vi "7813r01.vi"() -> ()   [LabVIEW 2018]
uses:
  <vilib>/Platform/TimedLoop/XDataNode/timing_clust.ctl
  <vilib>/Platform/TimedLoop/XDataNode/nitl_modes.ctl
  <vilib>/Platform/TimedLoop/XDataNode/wakeup.ctl
  <vilib>/rvi/Emulation/niFpgaGetClockAttributes.vi
  <vilib>/rvi/Emulation/niFpgaSctlEmulationGetInTimedLoop.vi
  <vilib>/rvi/Emulation/niFpgaEmulationReportErrorSimple.vi
  <vilib>/rvi/Emulation/niFpgaProcessEmulError.vi
  <vilib>/rvi/Emulation/niFpgaCriticalErrorInLSC.vi
  <vilib>/rvi/eio/common/nirviEmuTemplateMethod_errors.vi
  <vilib>/Platform/TimedLoop/XDataNode/XDataNode.xnode
  <vilib>/eio/EIONode/EIONode.xnode
  <vilib>/Platform/TimedLoop/XDataNode/XDNodeRunTimeDep.lvlib
panel:
  out "act":bool[](array[boolean])
  out "width":i32[](array[numeric])
  out "begin":i32[](array[numeric])
  in  "禁用shutup":bool
  in  "禁用trigger":bool
  out "T-run":bool
  in  "ShutUp":bool
  in  "Ready":bool
  in  "Abort":bool
  in  "max0+1":u32
  out "stop":bool
  in  "running":bool
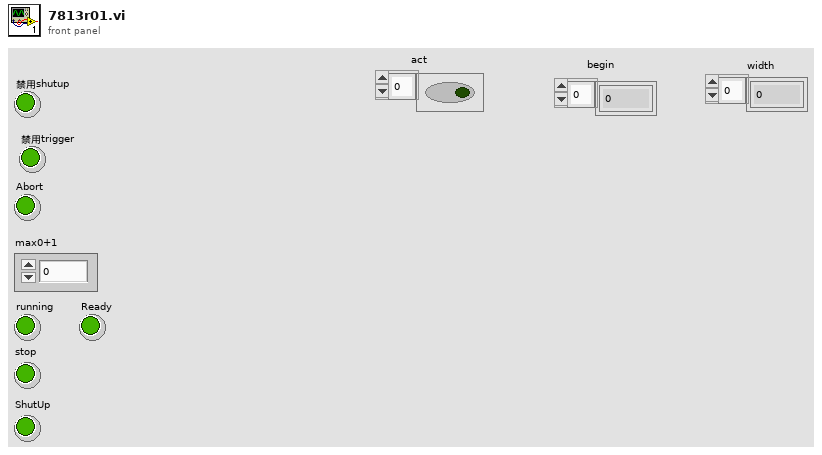
[diagram p1: front panel]
types:
  T1 = typedef "XDNodeRunTimeDep.lvlib/timing_clust.ctl" = cluster{"Expected End [f-1]":u64, "Actual End [f-1]":u64, "Finished Late? [f-1]":bool, "Expected End [i-1]":u64, "Actual End [i-1]":u64, "Finished Late? [i-1]":bool, "Expected Start [i]":u64, "Actual Start [i]":u64, "Expected Start [f]":u64, "Actual Start [f]":u64, "Source Name":string, "Structure Name":string, "Period":i64, "Deadline":i64, "Offset":i64, "Start":i64, "Priority":i32, "Timeout":i32, "Mode":T2, "Wakeup Reason":T3, "Error":errorcluster, "Source Type":string, "Secondary Source Type":string, "Global End Time":u64, "Global Start Time":u64, "Frame Duration":u64, "Iteration Duration":u64, "Assigned CPU":i32, "I/O Scan Engine Mode":u32}
  T2 = typedef "XDNodeRunTimeDep.lvlib/nitl_modes.ctl" = enum32{"No Change", "Process missed periods, maintain original phase", "Discard missed periods, maintain original phase", "Process missed periods, ignore original phase", "Discard missed periods, ignore original phase"}
  T3 = typedef "XDNodeRunTimeDep.lvlib/wakeup.ctl" = enum32{"Normal", "Aborted", "Asynchronous wakeup", "Timing source error", "Timed loop error", "Timeout"}
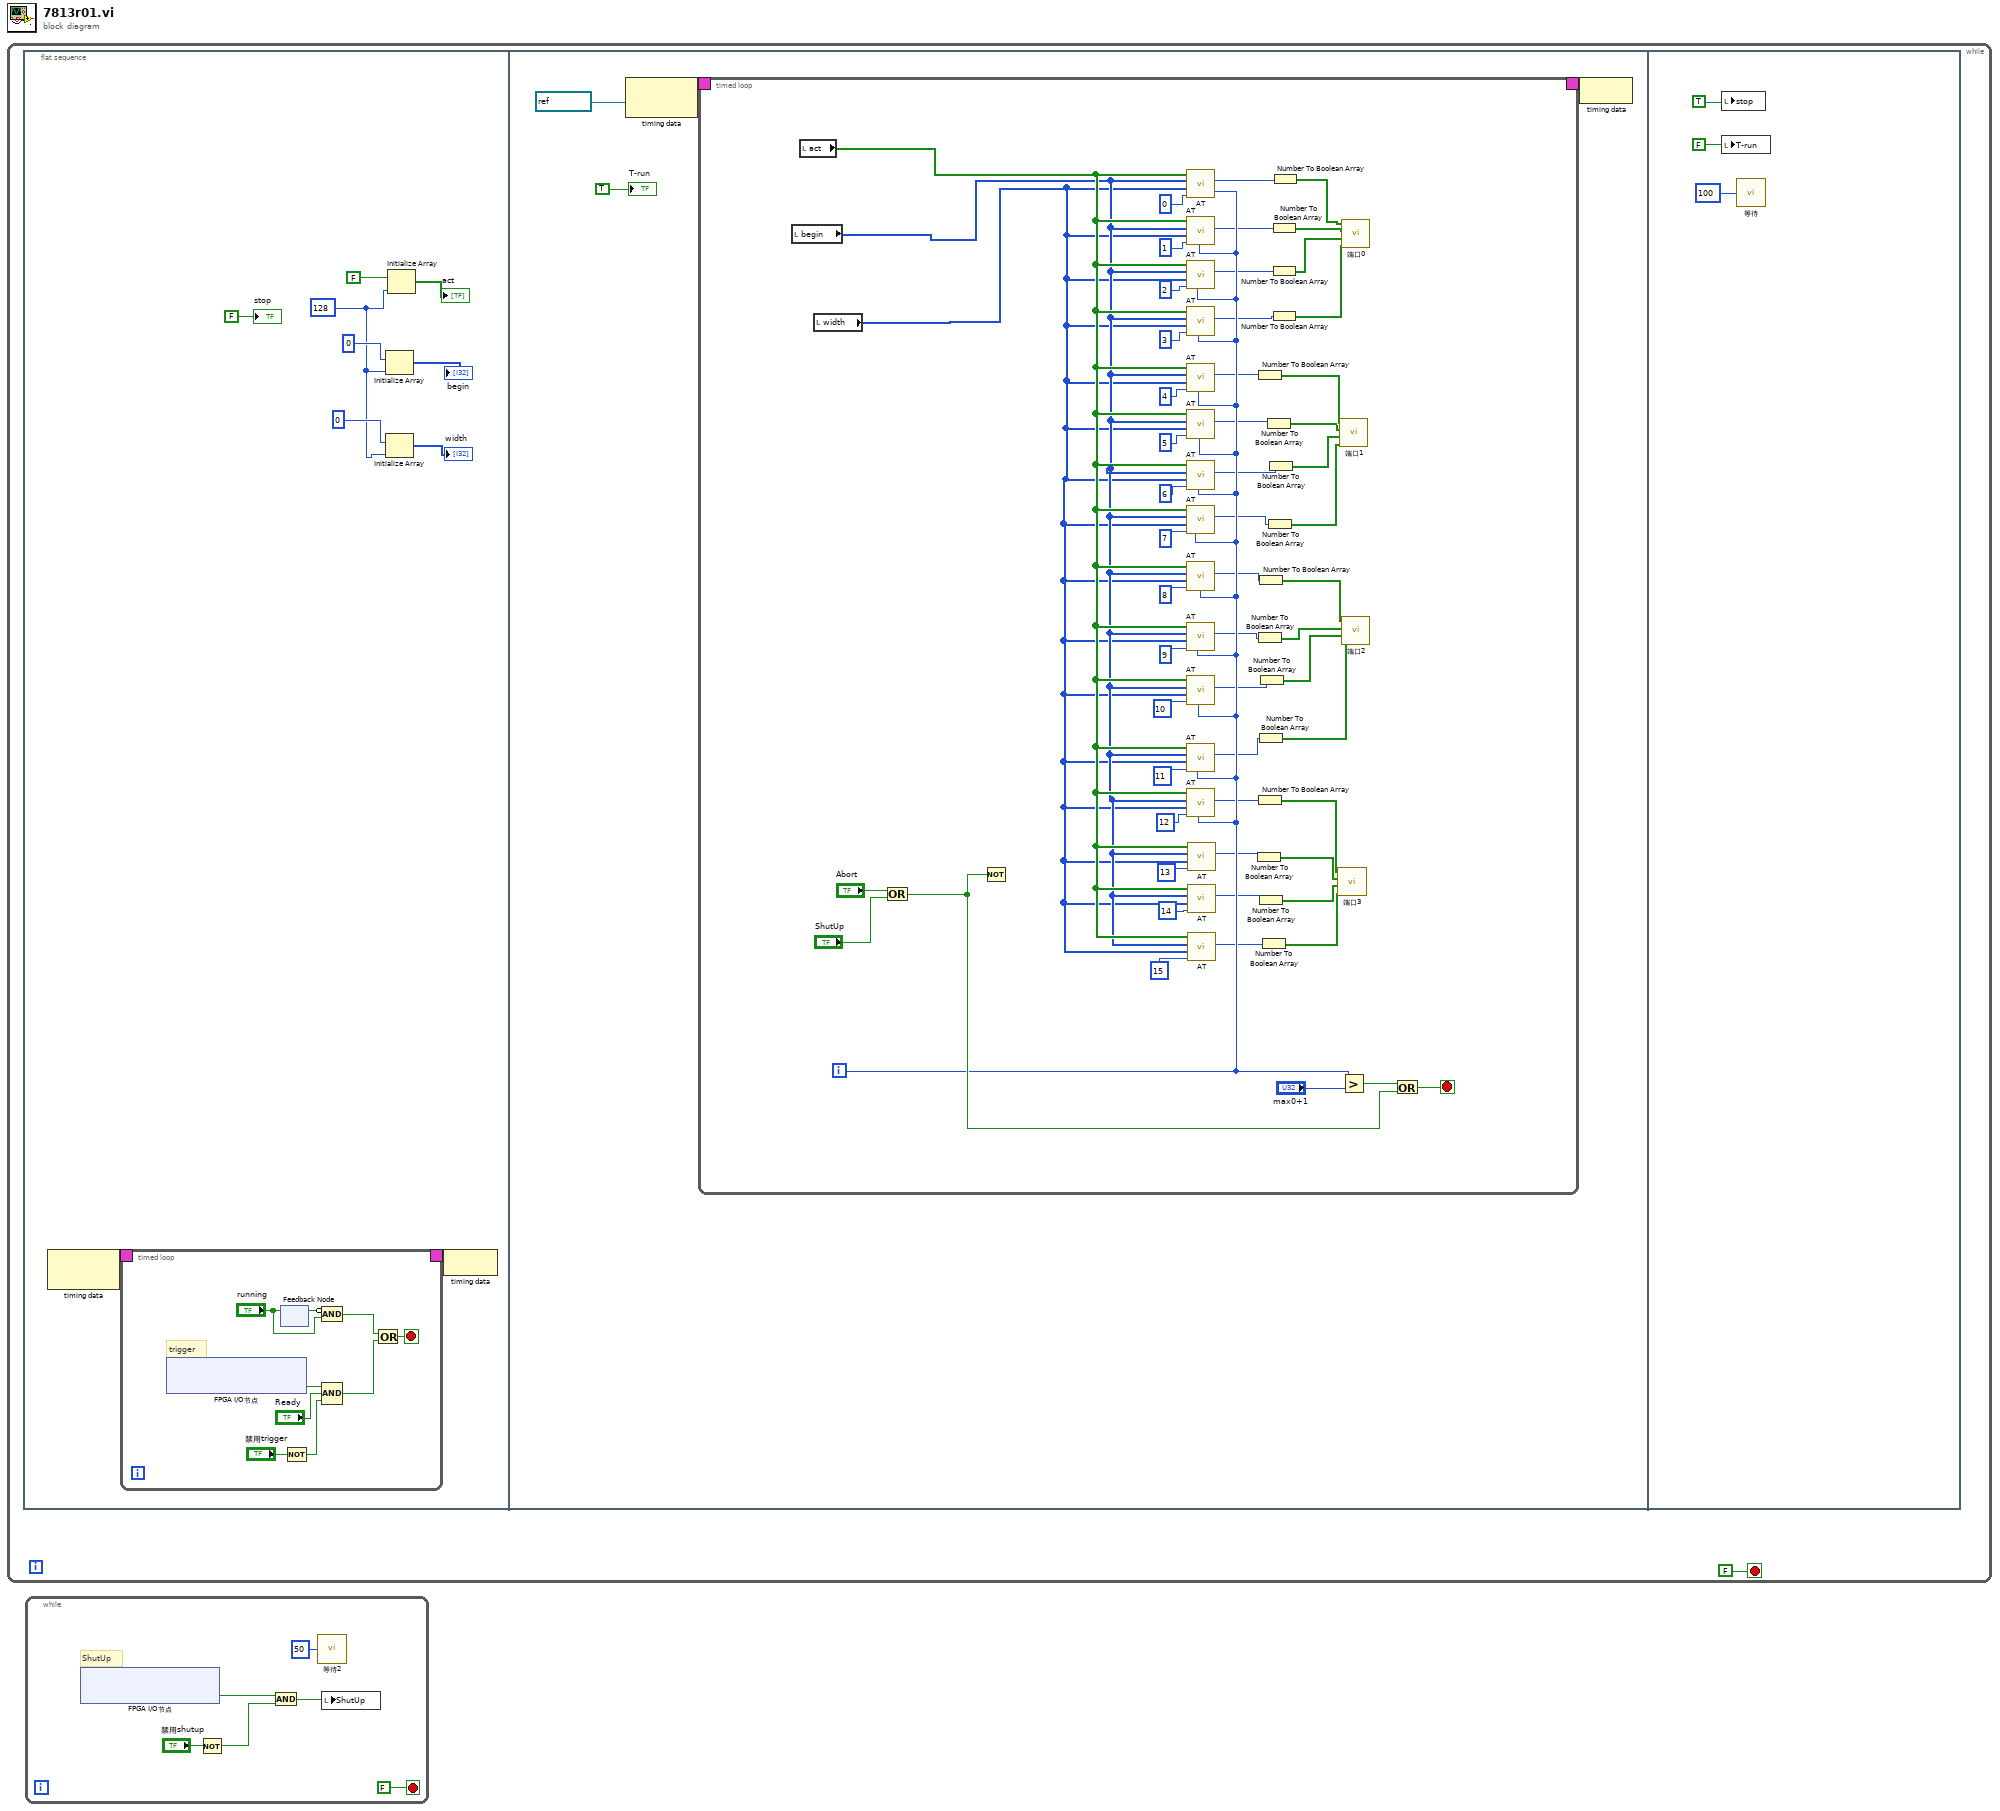
[diagram p0: block diagram]
diagram:
  n1 = while {
    stop <- FALSE stop-if-true
    n2 = flat-sequence {
      frame #0 {
        w2 = i16 128
        n3 = node-c288() -> (w11:T1)  [unwired: 1 in]
        n4 = timed-loop {
          timing: w11 -> [_]
          timing-out: [_] -> w10
          stop <- w19 stop-if-true
          # "trigger"
          n5 = xnode "FPGA I/O节点"() -> ("Connector0/DIO38"=w12:bool)  [unwired: 1 in, 1 out]
          n6 = feedback #1() -> (w15:bool)  [unwired: 1 in]
          n7 = feedback-in #1("running") -> ()
          n8 = Not(x="禁用trigger") -> (.not. x?=w16:bool)
          n9 = Compound Arithmetic op=AND(invert w15, "running") -> (w13:bool)
          n10 = Compound Arithmetic op=AND(w12, "Ready", w16) -> (w18:bool)
          n11 = Or(x=w13, y=w18) -> (x .or. y?=w19:bool)
        }
        n12 = Initialize Array(i16 0, w2) -> (→"begin":i16[])
        n13 = Initialize Array(i16 0, w2) -> (→"width":i16[])
        n14 = Initialize Array(FALSE, w2) -> (→"act":bool[])
        n15 = node-c288(w10) -> ()
        "stop" <- FALSE ("running")
      }
      frame #1 {
        n16 = node-c288(refnum<k21> "5MHz" ("源名称")) -> (w28:T1)
        n17 = timed-loop {
          timing: w28 -> [_]
          timing-out: [_] -> w27
          i -> [w67]
          stop <- w84 stop-if-true
          n18 = local read "begin"() -> (w62:i32[])
          n19 = local read "act"() -> (w63:bool[])
          n20 = local read "width"() -> (w61:i32[])
          n21 = Or(x="Abort", y="ShutUp") -> (x .or. y?=w83:bool)
          n22 = Not(x=w83) -> ()  [unwired: 1 out]
          n23 = call "AT.vi"("时间值"=w67, "数值"=i16 0, "width"=w61, "begin"=w62, "act"=w63) -> ("数字"=w60:u8)  [unwired: 6 in]
          n24 = call "AT.vi"("时间值"=w67, "数值"=i16 1, "width"=w61, "begin"=w62, "act"=w63) -> ("数字"=w59:u8)  [unwired: 6 in]
          n25 = call "AT.vi"("时间值"=w67, "数值"=i16 2, "width"=w61, "begin"=w62, "act"=w63) -> ("数字"=w58:u8)  [unwired: 6 in]
          n26 = call "AT.vi"("时间值"=w67, "数值"=i16 3, "width"=w61, "begin"=w62, "act"=w63) -> ("数字"=w57:u8)  [unwired: 6 in]
          n27 = call "AT.vi"("时间值"=w67, "数值"=i16 4, "width"=w61, "begin"=w62, "act"=w63) -> ("数字"=w52:u8)  [unwired: 6 in]
          n28 = call "AT.vi"("时间值"=w67, "数值"=i16 5, "width"=w61, "begin"=w62, "act"=w63) -> ("数字"=w51:u8)  [unwired: 6 in]
          n29 = call "AT.vi"("时间值"=w67, "数值"=i16 6, "width"=w61, "begin"=w62, "act"=w63) -> ("数字"=w50:u8)  [unwired: 6 in]
          n30 = call "AT.vi"("时间值"=w67, "数值"=i16 7, "width"=w61, "begin"=w62, "act"=w63) -> ("数字"=w49:u8)  [unwired: 6 in]
          n31 = call "AT.vi"("时间值"=w67, "数值"=i16 8, "width"=w61, "begin"=w62, "act"=w63) -> ("数字"=w44:u8)  [unwired: 6 in]
          n32 = call "AT.vi"("时间值"=w67, "数值"=i16 9, "width"=w61, "begin"=w62, "act"=w63) -> ("数字"=w43:u8)  [unwired: 6 in]
          n33 = call "AT.vi"("时间值"=w67, "数值"=i16 10, "width"=w61, "begin"=w62, "act"=w63) -> ("数字"=w42:u8)  [unwired: 6 in]
          n34 = call "AT.vi"("时间值"=w67, "数值"=i16 11, "width"=w61, "begin"=w62, "act"=w63) -> ("数字"=w41:u8)  [unwired: 6 in]
          n35 = call "AT.vi"("时间值"=w67, "数值"=i16 12, "width"=w61, "begin"=w62, "act"=w63) -> ("数字"=w36:u8)  [unwired: 6 in]
          n36 = call "AT.vi"("数值"=i16 13, "width"=w61, "begin"=w62, "act"=w63) -> ("数字"=w35:u8)  [unwired: 7 in]
          n37 = call "AT.vi"("数值"=i16 14, "width"=w61, "begin"=w62, "act"=w63) -> ("数字"=w34:u8)  [unwired: 7 in]
          n38 = call "AT.vi"("数值"=i16 15, "width"=w61, "begin"=w62, "act"=w63) -> ("数字"=w33:u8)  [unwired: 7 in]
          n39 = Number To Boolean Array(number=w35) -> (Boolean array=w31:bool[])
          n40 = Number To Boolean Array(number=w52) -> (Boolean array=w48:bool[])
          n41 = Number To Boolean Array(number=w43) -> (Boolean array=w39:bool[])
          n42 = Number To Boolean Array(number=w36) -> (Boolean array=w32:bool[])
          n43 = Number To Boolean Array(number=w44) -> (Boolean array=w40:bool[])
          n44 = Number To Boolean Array(number=w41) -> (Boolean array=w37:bool[])
          n45 = Number To Boolean Array(number=w34) -> (Boolean array=w30:bool[])
          n46 = Number To Boolean Array(number=w42) -> (Boolean array=w38:bool[])
          n47 = Number To Boolean Array(number=w33) -> (Boolean array=w29:bool[])
          n48 = Number To Boolean Array(number=w51) -> (Boolean array=w47:bool[])
          n49 = Number To Boolean Array(number=w49) -> (Boolean array=w45:bool[])
          n50 = Number To Boolean Array(number=w50) -> (Boolean array=w46:bool[])
          n51 = Number To Boolean Array(number=w59) -> (Boolean array=w55:bool[])
          n52 = Number To Boolean Array(number=w58) -> (Boolean array=w54:bool[])
          n53 = Number To Boolean Array(number=w57) -> (Boolean array=w53:bool[])
          n54 = Number To Boolean Array(number=w60) -> (Boolean array=w56:bool[])
          n55 = call "端口3.vi"("数组 4"=w29, "数组 3"=w30, "数组 2"=w31, "数组"=w32) -> ()  [unwired: 8 in]
          n56 = call "端口1.vi"("数组 4"=w45, "数组 3"=w46, "数组 2"=w47, "数组"=w48) -> ()  [unwired: 8 in]
          n57 = Greater?(x=w67, y="max0+1") -> (0:w85:bool)
          n58 = call "端口0.vi"("数组 4"=w53, "数组 3"=w54, "数组 2"=w55, "数组"=w56) -> ()  [unwired: 8 in]
          n59 = call "端口2.vi"("数组 4"=w37, "数组 3"=w38, "数组 2"=w39, "数组"=w40) -> ()  [unwired: 8 in]
          n60 = Or(x=w85, y=w83) -> (x .or. y?=w84:bool)
        }
        n61 = node-c288(w27) -> ()
        "T-run" <- TRUE ("T-run")
      }
      frame #2 {
        n62 = local write "stop"(TRUE ("running")) -> ()
        n63 = local write "T-run"(FALSE ("T-run")) -> ()
        n64 = call "等待"("Count(mSec)"=u32 100) -> ()  [unwired: 1 out]
      }
    }
  }
  n65 = while {
    stop <- FALSE stop-if-true
    # "ShutUp"
    n66 = xnode "FPGA I/O节点"() -> ("Connector0/DIO39"=w99:bool)  [unwired: 1 in, 1 out]
    n67 = Not(x="禁用shutup") -> (.not. x?=w100:bool)
    n68 = And(x=w99, y=w100) -> (x .and. y?=w101:bool)
    n69 = call "等待2"("Count(mSec)"=u32 50) -> ()  [unwired: 1 out]
    n70 = local write "ShutUp"(w101) -> ()
  }
